vi "Send and Receive.vi"(6 "timeout (ms) [500]":i32, 8 "error in (no error)":errorcluster, 9 "Data in":variant, 10 "Command in":string, 11 "Instrument in":refnum<class "Instrument.lvclass">) -> (0 "error out":errorcluster, 1 "Data out":variant, 2 "Command out":string, 3 "Instrument out":refnum<class "Instrument.lvclass">)   [LabVIEW 2019, in "Instrument.lvlib" / "Instrument.lvclass"]
doc: "Send and Receive remote messages to your Instrument instance.\n\n<b>Command</b> is a String\n\n<b>Data in</b> is a Variant containing your data payload. Typically the transport layer will format this data how it wishes (e.f. RemoteControl.ZMQ will create a JSON-RPC request object)\n\n<b>Data out</b> will be formatted by the remote Instrument and/or transport layer and you will need to convert it to LVdata later"
uses:
  Instrument.lvclass
  Instrument.lvclass/Instrument.ctl
  <userlib>/LevyLab/RemoteControl/RemoteControl.lvclass
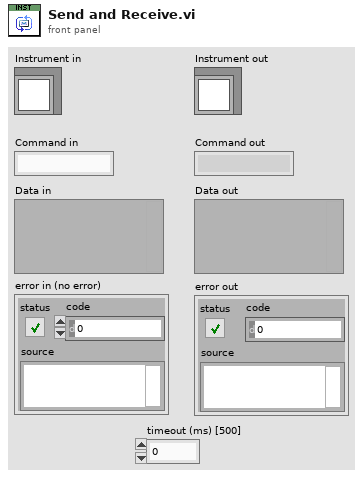
[diagram p1: front panel]
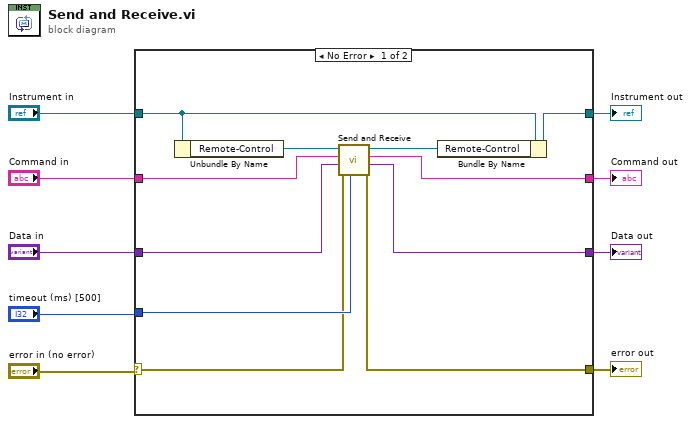
[diagram p0: block diagram]
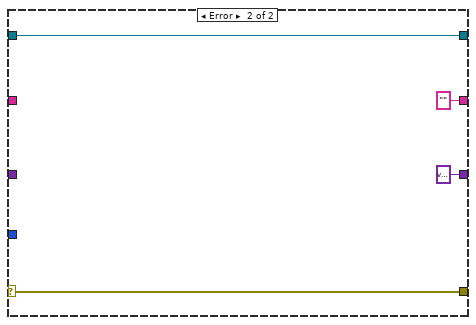
[diagram p2: hidden frame]
diagram:
  n1 = case shown="No Error" "error in (no error)" {
    selector: "error in (no error)" -> [w11 w24]
    tunnel: "Instrument in" -> [w14 w23]
    tunnel: "timeout (ms) [500]" -> [w20 _]
    tunnel: "Data in" -> [w19 _]
    tunnel: "Command in" -> [w13 _]
    tunnel: [w15 w23] -> w5
    tunnel: [w10 w24] -> w4
    tunnel: [w12 "" ("Command out")] -> w3
    tunnel: [w18 variant ("Data out")] -> w2
    frame No Error {
      n2 = Unbundle By Name(w14) -> ("Remote-Control"=w17:refnum<class "RemoteControl.lvclass">)
      n3 = call <userlib>:"Send and Receive.vi"("timeout (ms) [500]"=w20, "error in (no error)"=w11, "Data"=w19, "Command"=w13, "RemoteControl in"=w17) -> ("error out"=w10:errorcluster, "Data out"=w18:variant, "Command out"=w12:string, "RemoteControl out"=w16:refnum<class "RemoteControl.lvclass">)  [unwired: 3 in]
      n4 = Bundle By Name(cluster=w14, "Remote-Control"=w16) -> (w15:refnum<class "Instrument.lvclass">)
    }
    frame Error {
    }
  }
  "Data out" <- w2
  "error out" <- w4
  "Command out" <- w3
  "Instrument out" <- w5
